vi "Configure Attenuator.vi"(5 "Use Eletronic Attenuator (F)":bool, 7 "Auto Attenuator (T)":bool=TRUE, 8 "error in (no error)":errorcluster, 10 "Attenuator (dB)":u32, 11 "SA-FSW in":refnum<class "SA-FSW.lvclass">) -> (0 "error out":errorcluster, 3 "SA-FSW out":refnum<class "SA-FSW.lvclass">)   [LabVIEW 2020, in "SA-FSW.lvclass"]
uses:
  SA-FSW.lvclass
  C:/Sandbox/Git_Sandbox/WiSpry Test Framework source code (LV20)/WiSpry Test Framework/Instruments/Instrument.lvclass
  C:/Sandbox/Git_Sandbox/WiSpry Test Framework source code (LV20)/WiSpry Test Framework/Instruments/Spectrum Analyzer/Spectrum Analyzer.lvclass
  Instrument.lvclass/Instrument.ctl
  Spectrum Analyzer.lvclass/Spectrum Analyzer.ctl
  Instrument.lvclass
  Spectrum Analyzer.lvclass
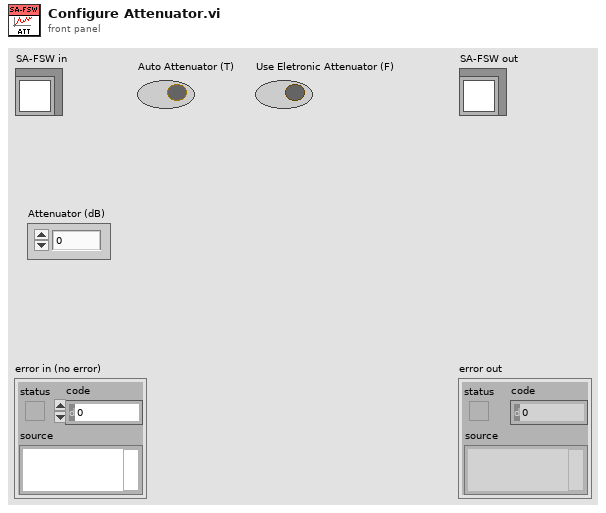
[diagram p1: front panel]
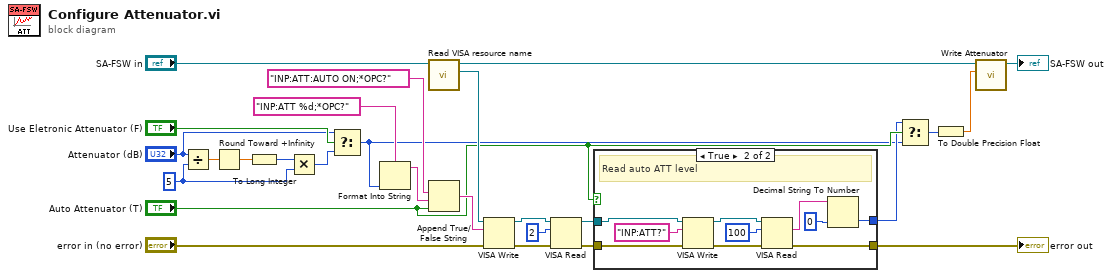
[diagram p0: block diagram]
diagram:
  w3 = u32 5 ("y")
  n1 = Divide(x="Attenuator (dB)", y=w3) -> (x/y=w5:dbl)
  n2 = Round Toward +Infinity(x=w5) -> (ceil(x): smallest int >= x=w4:dbl)
  n3 = To Long Integer(number=w4) -> (32bit integer=w2:i32)
  n4 = Multiply(x=w2, y=w3) -> (x*y=w1:u32)
  n5 = Select(t="Attenuator (dB)", s="Use Eletronic Attenuator (F)", f=w1) -> (s? t:f=w7:u32)
  n6 = Format Into String(format string="INP:ATT %d;*OPC?", w7) -> (resulting string=w19:string)  [unwired: 2 in, 1 out]
  n7 = call "Read VISA resource name.vi"("Instrument in"="SA-FSW in") -> ("VISA resource name"=w26:refnum<visa-resource-name>, "Instrument out"=w21:refnum<class "SA-FSW.lvclass">)  [unwired: 9 in]
  n8 = Append True/False String(1:"Auto Attenuator (T)", 2:w19, 3:"INP:ATT:AUTO ON;*OPC?" ("true string")) -> (0:w17:string)  [unwired: 1 in]
  n9 = VISA Write(VISA resource name=w26, write buffer=w17, error in (no error)="error in (no error)") -> (VISA resource name out=w23:refnum<visa-resource-name>, error out=w24:errorcluster)  [unwired: 1 out]
  n10 = VISA Read(VISA resource name=w23, byte count=u32 2, error in (no error)=w24) -> (VISA resource name out=w15:refnum<visa-resource-name>, error out=w16:errorcluster)  [unwired: 2 out]
  n11 = case shown="True" "Auto Attenuator (T)" {
    tunnel: w16 -> [w28 w38]
    tunnel: w15 -> [_ w37]
    tunnel: [w28 w31] -> w14
    tunnel: [_ w30] -> w11
    frame False {
    }
    frame True {
      # "Read auto ATT level"
      n12 = VISA Write(VISA resource name=w37, write buffer="INP:ATT?", error in (no error)=w38) -> (VISA resource name out=w34:refnum<visa-resource-name>, error out=w35:errorcluster)  [unwired: 1 out]
      n13 = VISA Read(VISA resource name=w34, byte count=u32 100, error in (no error)=w35) -> (read buffer=w32:string, error out=w31:errorcluster)  [unwired: 2 out]
      n14 = Decimal String To Number(string=w32, default (0L)=u32 0) -> (number=w30:u32)  [unwired: 1 in, 1 out]
    }
  }
  "error out" <- w14
  n15 = Select(t=w11, s="Auto Attenuator (T)", f=w7) -> (s? t:f=w12:u32)
  n16 = To Double Precision Float(number=w12) -> (double precision float=w10:dbl)
  n17 = call "Write Attenuator.vi"("Attenuator"=w10, "Spectrum Analyzer in"=w21) -> ("Spectrum Analyzer out"=→"SA-FSW out":refnum<class "SA-FSW.lvclass">)  [unwired: 9 in]
